vi "lvEtherbone.application_example.vi"() -> ()   [LabVIEW 2012, in "lvEtherbone.lvlib"]
doc: "This example \"getting started\" performs a write and then a read via Etherbone.\n\nFor using this example, you need a Etherbone device. In case you don't have one at hand, try\n\n\"eb-snoop 5555 0x10000-0x20000\" from the command line\n\non your machine."
uses:
  lvEtherbone.lvlib
panel:
  out "data_out":u32 format="%.0x"
  in  "address_read":u32=65536 format="%.0x"
  out "device_id":u32=3284528890 format="%.0x"
  out "vendor_id":u64=1617 format="%.0x"
  out "addr_last":u64=131072 format="%.0x"
  out "addr_first":u64=65536 format="%.0x"
  out "name":string="Software-Memory    "
  in  "data_write":u32=4660 format="%.0x"
  in  "address_write":u32=65536 format="%.0x"
  in  "address":string="udp/localhost/5555"
  out "error out":errorcluster
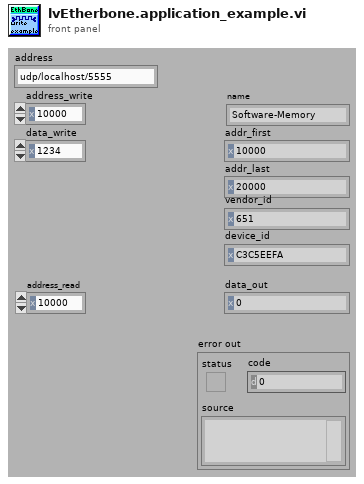
[diagram p1: front panel]
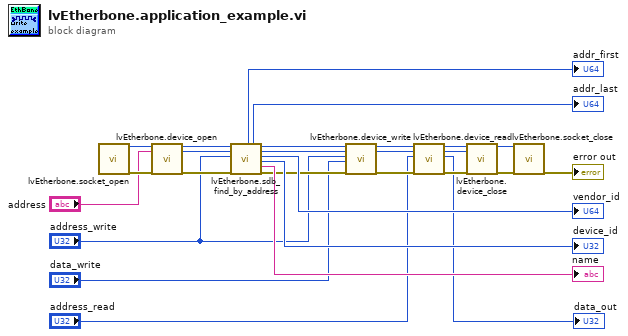
[diagram p0: block diagram]
diagram:
  n1 = call "lvEtherbone.socket_open.vi"() -> ("eb_socket_ID"=w26:i32, "error out"=w25:errorcluster)  [unwired: 17 in, 1 out]
  n2 = call "lvEtherbone.device_open.vi"("eb_socket_ID"=w26, "address"="address", "error in (no error)"=w25) -> ("eb_socket_ID out"=w21:i32, "eb_device_ID"=w20:i32, "error out"=w19:errorcluster)  [unwired: 13 in, 1 out]
  n3 = call "lvEtherbone.sdb_find_by_address.vi"("eb_socket_ID"=w21, "eb_device_ID"=w20, "address"="address_write", "error in (no error)"=w19) -> ("addr_first"=→"addr_first":u64, "addr_last"=→"addr_last":u64, "eb_socket_ID out"=w13:i32, "eb_device_ID out"=w11:i32, "vendor_id"=→"vendor_id":u64, "device_id"=→"device_id":u32, "name"=→"name":string, "error out"=w12:errorcluster)  [unwired: 7 in, 1 out]
  n4 = call "lvEtherbone.device_write.vi"("eb_socket_ID"=w13, "eb_device_ID"=w11, "address"="address_write", "data"="data_write", "error in (no error)"=w12) -> ("eb_socket_ID out"=w8:i32, "eb_device_ID out"=w7:i32, "error out"=w6:errorcluster)  [unwired: 11 in, 1 out]
  n5 = call "lvEtherbone.device_read.vi"("eb_socket_ID"=w8, "eb_device_ID"=w7, "address"="address_read", "error in (no error)"=w6) -> ("eb_socket_ID out"=w5:i32, "eb_device_ID out"=w4:i32, "data"=→"data_out":u32, "error out"=w3:errorcluster)  [unwired: 11 in, 1 out]
  n6 = call "lvEtherbone.device_close.vi"("eb_socket_ID"=w5, "eb_device_ID"=w4, "error in (no error)"=w3) -> ("eb_socket_ID out"=w23:i32, "error out"=w22:errorcluster)  [unwired: 14 in, 1 out]
  n7 = call "lvEtherbone.socket_close.vi"("eb_socket_ID"=w23, "error in (no error)"=w22) -> ("error out"=→"error out":errorcluster)  [unwired: 16 in, 1 out]
